vi "tuning_test.vi"() -> ()   [LabVIEW 2011]
panel:
  out "XY Graph":cluster{i32[], dbl[]}(graph)
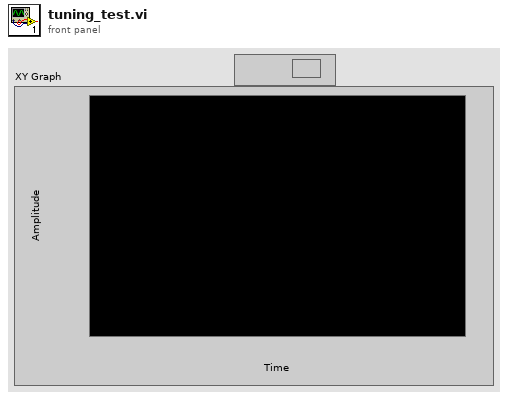
[diagram p1: front panel]
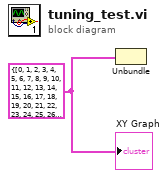
[diagram p0: block diagram]
diagram:
  w1 = cluster{i32[], dbl[]} {[0, 1, 2, 3, 4, 5, 6, 7, 8, 9, 10, 11, 12, 13, 14, 15, 16, 17, 18, 19, 20, 21, 22, 23, 24, 25, 26, 27, 28, 29, 30, 31, 32, 33, 34, 35, 36, 37, 38, 39, 40, 41, 42, 43, 44, 45, 46, 47, 48, 49, 50, 51, 52, 53, 54, 55, 56, 57, 58, 59, 60, 61, 62, 63, 64, 65, 66, 67, 68, 69, 70, 71, 72, 73, 74, 75, 76, 77, 78, 79, 80, 81, 82, 83, 84, 85, 86, 87, 88, 89, 90, 91, 92, 93, 94, 95, 96, 97, 98, 99, 100, 101, 102, 103, 104, 105, 106, 107, 108, 109, 110, 111, 112, 113, 114, 115, 116, 117, 118, 119, 120, 121, 122, 123, 124, 125, 126, 127, 128, 129, 130, 131, 132, 133, 134, 135, 136, 137, 138, 139, 140, 141, 142, 143, 144, 145, 146, 147, 148, 149, 150, 151, 152, 153, 154, 155, 156, 157, 158, 159, 160, 161, 162, 163, 164, 165, 166, 167, 168, 169, 170, 171, 172, 173, 174, 175, 176, 177, 178, 179, 180, 181, 182, 183, 184, 185, 186, 187, 188, 189, 190, 191, 192, 193, 194, 195, 196, 197, 198, 199, 200, 201, 202, 203, 204, 205, 206, 207, 208, 209, 210, 211, 212, 213, 214, 215, 216, 217, 218, 219, 220, 221, 222, 223, 224, 225, 226, 227, 228, 229, 230, 231, 232, 233, 234, 235, 236, 237, 238, 239, 240, 241, 242, 243, 244, 245, 246, 247, 248, 249, 250, 251, 252, 253, 254, 255, 256, 257, 258, 259, 260, 261, 262, 263, 264, 265, 266, 267, 268, 269, 270, 271, 272, 273, 274, 275, 276, 277, 278, 279, 280, 281, 282, 283, 284, 285, 286, 287, 288, 289, 290, 291, 292, 293, 294, 295, 296, 297, 298, 299, 300, 301, 302, 303, 304, 305, 306, 307, 308, 309, 310, 311, 312, 313, 314, 315, 316, 317, 318, 319, 320, 321, 322, 323, 324, 325, 326, 327, 328, 329, 330, 331, 332, 333, 334, 335, 336, 337, 338, 339, 340, 341, 342, 343, 344, 345, 346, 347, 348, 349, 350, 351, 352, 353, 354, 355, 356, 357, 358, 359, 360, 361, 362, 363, 364, 365, 366, 367, 368, 369, 370, 371, 372, 373, 374, 375, 376, 377, 378, 379, 380, 381, 382, 383, 384, 385, 386, 387, 388, 389, 390, 391, 392, 393, 394, 395, 396, 397, 398, 399, 400, 401, 402, 403, 404, 405, 406, 407, 408, 409, 410, 411, 412, 413, 414, 415, 416, 417, 418, 419, 420, 421, 422, 423, 424, 425, 426, 427, 428, 429, 430, 431, 432, 433, 434, 435, 436, 437, 438, 439, 440, 441, 442, 443, 444, 445, 446, 447, 448, 449, 450, 451, 452, 453, 454, 455, 456, 457, 458, 459, 460, 461, 462, 463, 464, 465, 466, 467, 468, 469, 470, 471, 472, 473, 474, 475, 476, 477, 478, 479, 480, 481, 482, 483, 484, 485, 486, 487, 488, 489, 490, 491, 492, 493, 494, 495, 496, 497, 498, 499, 500, 501, 502, 503, 504, 505, 506, 507, 508, 509, 510, 511, 512, 513, 514, 515, 516, 517, 518, 519, 520, 521, 522, 523, 524, 525, 526, 527, 528, 529, 530, 531, 532, 533, 534, 535, 536, 537, 538, 539, 540, 541, 542, 543, 544, 545, 546, 547, 548, 549, 550, 551, 552, 553, 554, 555, 556, 557, 558, 559, 560, 561, 562, 563, 564, 565, 566, 567, 568, 569, 570, 571, 572, 573, 574, 575, 576, 577, 578, 579, 580, 581, 582, 583, 584, 585, 586, 587, 588, 589, 590, 591, 592, 593, 594, 595, 596, 597, 598, 599, 600, 601, 602, 603, 604, 605, 606, 607, 608, 609, 610, 611, 612, 613, 614, 615, 616, 617, 618, 619, 620, 621, 622, 623, 624, 625, 626, 627, 628, 629, 630, 631, 632, 633, 634, 635, 636, 637, 638, 639, 640, 641, 642, 643, 644, 645, 646, 647, 648, 649, 650, 651, 652, 653, 654, 655, 656, 657, 658, 659, 660, 661, 662, 663, 664, 665, 666, 667, 668, 669, 670, 671, 672, 673, 674, 675, 676, 677, 678, 679, 680, 681, 682, 683, 684, 685, 686, 687, 688, 689, 690, 691, 692, 693, 694, 695, 696, 697, 698, 699, 700, 701, 702, 703, 704, 705, 706, 707, 708, 709, 710, 711, 712, 713, 714, 715, 716, 717, 718, 719], [0.005163496779999999, 0.005067374419, 0.005019692889999998, 0.004978500865999999, 0.0049584110729999995, 0.00494455779, 0.004903066485, 0.004896530929, 0.004880330292, 0.004855177923999999, 0.0047993269750000005, 0.0046631170910000005, 0.004542808654000001, 0.004450621223, 0.004386301712, 0.00432218942, 0.004258146137000001, 0.004217115137, 0.0041646011169999995, 0.004128793907, 0.004072965913999999, 0.004036284378999999, 0.004002226237999999, 0.003977994153, 0.003909670723999999, 0.003839253053, 0.003779075738, 0.003699775296, 0.0036282991290000005, 0.0035629671070000007, 0.0034715622649999995, 0.003404113207, 0.003354659746, 0.0033112354810000003, 0.0032005922650000006, 0.003136986193, 0.00301980749, 0.0029431304430000004, 0.0028419683679999997, 0.002778316312, 0.002698302478, 0.0026508510799999998, 0.002591755498, 0.002476762958, 0.002406690456, 0.002356040384, 0.0023017082590000002, 0.002219623326, 0.0021449944, 0.0020812042740000003, 0.002020704862, 0.001944258006, 0.0018612755710000002, 0.001797554502, 0.0017389191200000002, 0.0016755202440000001, 0.001597784644, 0.001522603363, 0.0014572023889999999, 0.001393688319, 0.0013246974999999999, 0.001252392749, 0.0011796738609999998, 0.00110727715, 0.00104031133, 0.0009799039515, 0.0009230175054000001, 0.0008696749981, 0.0008188407983999999, 0.0007630129285000001, 0.0007079674803999999, 0.0006573633814, 0.0006091065414, 0.0005715965176, 0.0005455925944, 0.0005262162478000002, 0.0005116264509000001, 0.0004915136727, 0.00046408299230000003, 0.0004366523296, 0.00042381145470000005, 0.0004150437628, 0.0003989581746, 0.000375784759, 0.00034384366010000003, 0.00030764528780000003, 0.00027413941000000005, 0.0002414158765, 0.0002199223687, 0.0002098199273, 0.00021005008180000002, 0.00021156888669999997, 0.00021182201900000002, 0.0002084162045, 0.0002094287224, 0.00021014211380000004, 0.0002181274147, 0.00022921935309999997, 0.00023499543020000002, 0.00023973596109999997, 0.0002453969951, 0.0002538885048, 0.0002666143584, 0.0002948734793, 0.0003390800908, 0.0003910879545, 0.0004366983632, 0.00047275868710000004, 0.0005059883988, 0.0005384818010999999, 0.0005604355597, 0.0005781550134, 0.0005994874285, 0.0006350644282999999, 0.0006777292814999999, 0.0007130301907, 0.0007522661879, 0.0008017426417, 0.0008465476624000001, 0.0008945282665999999, 0.0009516218445, 0.0010136170074, 0.001077591267, 0.0011420027110000002, 0.001207771943, 0.001281549398, 0.0013521281650000002, 0.001426711048, 0.001501409012, 0.0015786613930000002, 0.0016642902170000001, 0.001764876955, 0.001854556053, 0.0019330509819999997, 0.001988441614, 0.00206979015, 0.002169617591, 0.002259664702, 0.0023309569119999997, 0.002392123616, 0.002458721283, 0.002527873357, 0.00262843708, 0.002727988362, 0.002846892923, 0.002969203446, 0.0030465937679999998, 0.003119519911, 0.0031939186620000004, 0.0032623112420000003, 0.0033096936300000004, 0.003375554829, 0.0034586063109999995, 0.003576659433, 0.0036718844429999994, 0.003751437995, 0.003836882673, 0.003914204169, 0.0039525425990000005, 0.003981192829, 0.004038470564999999, 0.004073679541, 0.00410115607, 0.004147710045, 0.0041927452670000006, 0.004247215295999999, 0.004309003288, 0.0043698708999999995, 0.00441168435, 0.004466361599, 0.004509693895000001, 0.004537032589, 0.004605563264, 0.00467890352, 0.004729944886000001, 0.004770423472, 0.0047632667250000005, 0.004818588309, 0.0048896042619999995, 0.004951392302, 0.005038793154, 0.005045282606999999, 0.005042152991, 0.0050377344239999995, 0.0050650041549999995, 0.005108750517, 0.005150540779999999, 0.005148584815, 0.0051888794160000005, 0.005234305656000001, 0.005266131739999999, 0.00529043288, 0.005290870042, 0.005267558526000001, 0.005254533513999999, 0.005249194707999999, 0.00528870672, 0.005303756894, 0.0053155161440000005, 0.005309855147999999, 0.005336917751, 0.005349045108, 0.005311903311, 0.005294805067, 0.005262058507, 0.005250529385000001, 0.0052575481139999995, 0.005224502552000001, 0.005146951043, 0.005057778255, 0.004995622066999999, 0.004946490797, 0.004906219151, 0.004888568586, 0.004888361552999999, 0.004896485014, 0.0048900875270000005, 0.004875382596, 0.004836514871, 0.004757490522, 0.00467503746, 0.004597578103999999, 0.004487878130999999, 0.004384138528, 0.004336963361, 0.0043169425319999994, 0.004281457513, 0.004219807636, 0.004116298118, 0.004016700945, 0.003940990356, 0.0038744617960000003, 0.0038080253429999995, 0.0037455238859999997, 0.003657731948, 0.003582619737, 0.0035078526250000006, 0.0034235816210000007, 0.0033413816000000007, 0.0032778216060000004, 0.003217046055, 0.003170722258, 0.0031204172869999996, 0.003048411825, 0.002945592673, 0.002855016361, 0.0027618854760000006, 0.0026850243569999997, 0.002612581617, 0.00253312008, 0.00246613128, 0.0024227760489999996, 0.002364439843, 0.0023274590500000003, 0.0022610685320000002, 0.002164946101, 0.002067350922, 0.0019887407769999996, 0.001923454867, 0.001850229654, 0.0017620695070000001, 0.001694459374, 0.0016268951480000002, 0.0015538541120000001, 0.001474392554, 0.001410556398, 0.001351690911, 0.001288291966, 0.001230554061, 0.001174427126, 0.0011069089519999999, 0.001031727705, 0.0009569837246000001, 0.0008908923716, 0.0008290122205, 0.0007700086863, 0.0007149171957999999, 0.0006650035096, 0.0006183804945000001, 0.0005712513230000001, 0.0005292768591000001, 0.0004940450628, 0.0004643591412, 0.0004372506374, 0.00041294963459999996, 0.0003859331977, 0.0003572828487, 0.0003281262587, 0.00029933788179999993, 0.0002788108745, 0.00026277128490000004, 0.00024406230079999998, 0.0002255373766, 0.00020860031510000002, 0.0001933201508, 0.00017527848540000005, 0.00016823673240000002, 0.0001699626187, 0.0001768203073, 0.0001852888322, 0.0001904666091, 0.00019161723450000003, 0.0001907887724, 0.0001927218181, 0.0001992112841, 0.00020358363099999996, 0.00021398521350000002, 0.00022770054620000003, 0.0002466166451, 0.00026771892710000003, 0.0002917667937, 0.00031986484809999995, 0.0003460528416000001, 0.00037293126220000006, 0.0004022719369, 0.0004359389509, 0.00047720006849999994, 0.0005206933186999999, 0.0005615861563000001, 0.0006020648232, 0.0006502986243999999, 0.0007099005335, 0.0007726551091000001, 0.0008327862946999999, 0.0008956559586000001, 0.0009586866014999999, 0.001016723679, 0.0010723444630000001, 0.0011222811769999999, 0.001164969021, 0.0012200374510000001, 0.0012946433980000002, 0.00137817806, 0.001445811289, 0.0015114884359999998, 0.001574979397, 0.001653060223, 0.001743268442, 0.0018260437180000002, 0.001895034629, 0.001958824833, 0.00203018596, 0.002105229162, 0.002169778616, 0.002219945472, 0.002265348843, 0.0023174947370000003, 0.002397439465, 0.002500258503, 0.002580778578, 0.0026439934290000003, 0.0027078756369999994, 0.0028000168490000003, 0.0028692149090000004, 0.0029648310740000004, 0.0030518636099999994, 0.0031166893659999996, 0.0031846676739999994, 0.0032518175889999995, 0.003347433826, 0.003455821797, 0.003553877281, 0.003617621354, 0.003675336319999999, 0.00374349875, 0.0038037910130000003, 0.003868041328999999, 0.003943475755, 0.004014146561999999, 0.004046340846, 0.004107139305, 0.0041663730509999995, 0.0042568343699999995, 0.004356063435999999, 0.0044169541909999995, 0.0044630248559999995, 0.004542509419, 0.004655016772000001, 0.004711304979, 0.004742808825, 0.004761793882000001, 0.0047857495969999995, 0.004832510696000001, 0.00492881732, 0.0049911807310000006, 0.0050461341630000005, 0.005067282403000001, 0.005071516567000001, 0.00507338061, 0.005063347284, 0.005069054336, 0.005091767478, 0.005116666806, 0.005122028617, 0.005140737817, 0.005161931925000001, 0.005183379492, 0.005233638315, 0.005237021204, 0.005229266126999999, 0.005247606896999999, 0.005280261392, 0.0052912842039999994, 0.005279778131, 0.005226550624, 0.005188304094, 0.005178178661, 0.0051268381989999995, 0.005104355094, 0.005108704605, 0.005076901521, 0.005056282458999999, 0.005045949994, 0.004990398185, 0.004914710716999999, 0.004886566662, 0.004869537615, 0.004838931233999999, 0.004827125882999999, 0.004853613023, 0.004844177930999999, 0.0048127660039999996, 0.004760919464, 0.004721683404, 0.004676740431, 0.004602088361, 0.004554452888000001, 0.004508612305000001, 0.004448849336, 0.004371596872, 0.004298141598, 0.004235801287, 0.004205908252, 0.004187636310000001, 0.0041415197299999994, 0.004125963336, 0.004063507961, 0.003969249547, 0.0038744617950000003, 0.003814123547, 0.0037748644130000003, 0.0036916290170000005, 0.0036297949269999998, 0.003543337715, 0.0034873716999999998, 0.003408899716, 0.0033433146770000003, 0.0032485729079999998, 0.0031890631200000006, 0.00310387148, 0.0030086235609999997, 0.00292709088, 0.002862150221, 0.002791617323, 0.002713996939, 0.0026494703480000005, 0.0025744732, 0.0024894427510000006, 0.002392468835, 0.002292365233, 0.002199303521, 0.002107852535, 0.002036353295, 0.001962161554, 0.0018770160160000004, 0.001794470871, 0.0017097855120000002, 0.001611223816, 0.001543613592, 0.00148196359, 0.001423236228, 0.001358341518, 0.001293032534, 0.001222062565, 0.001159607119, 0.0010932856929999999, 0.0010236963872, 0.0009635652298000001, 0.0009028587725, 0.000857639557, 0.0008077258304000001, 0.0007566845511000001, 0.0007070009772, 0.0006628863455, 0.0006217633317, 0.0005855880094999999, 0.0005464441142, 0.0005036641901, 0.00046233404729999997, 0.0004282298411, 0.00039603559980000007, 0.0003605506209, 0.00032757394370000004, 0.000304515616, 0.00028373550739999997, 0.0002713549037, 0.0002596646256, 0.0002497693291, 0.0002355247037, 0.0002155960598, 0.00019587451529999998, 0.0001770734408, 0.000159054788, 0.0001439126571, 0.00013440858750000002, 0.0001292998684, 0.00012545681080000003, 0.000125709966, 0.00012743586850000001, 0.00013588138679999998, 0.0001566384904, 0.0001995334691, 0.00025066682289999996, 0.0002854384305, 0.0003082436045, 0.0003360424948, 0.00036229956, 0.000381583866, 0.0004054016084000001, 0.0004310603923, 0.0004553843549, 0.00048244685159999997, 0.0005036872405, 0.0005258480787000001, 0.0005511846274999999, 0.0005961046437999999, 0.0006541646784999999, 0.0007094862638, 0.0007599062577000001, 0.0008092907257000001, 0.0008690306511000001, 0.0009344316145, 0.0009934812493, 0.0010433259299999999, 0.001086013754, 0.001130910742, 0.0011782931620000002, 0.0012328553359999999, 0.001308726915, 0.001378408237, 0.001444637638, 0.0015097855019999998, 0.0015721488500000003, 0.001642727667, 0.00171065994, 0.0017643017220000002, 0.001836790504, 0.0019079906049999998, 0.001984391478, 0.002053635497, 0.0021220741330000006, 0.002211799169, 0.0022944133749999997, 0.0023712745169999997, 0.0024567881589999995, 0.002509371379, 0.002560458681, 0.0026346044139999997, 0.0027116956900000004, 0.002782550501, 0.002870526583, 0.002963358327, 0.0030565351929999996, 0.0031379067329999994, 0.0032162407179999997, 0.0032958402300000003, 0.003362207835, 0.003419692513, 0.0034609535930000004, 0.0035358586589999998, 0.0036595038600000006, 0.0037571680260000003, 0.003812420623999999, 0.003873633384, 0.0039343629050000006, 0.004006299377, 0.0040949428449999995, 0.004153969373, 0.004222154711, 0.004285415634, 0.0043417268920000005, 0.004374473357, 0.004444177728, 0.0045582499350000005, 0.0046384708939999995, 0.0046693995129999995, 0.00467989319, 0.004701041338000001, 0.004724030662, 0.004774105594000001, 0.004809222417000001, 0.004851127648, 0.004924030649, 0.0049912726049999995, 0.005023006677, 0.005077914055999999, 0.005120693984, 0.005134317186, 0.005104194067999999, 0.005083690072, 0.00509416056, 0.005126377987, 0.005150586879000001, 0.005199188876999999, 0.005219301722, 0.005296830229, 0.005336526360999999, 0.005388143099999999, 0.005415435507, 0.005421695065000001, 0.005405218294999999, 0.005341404956, 0.005274968455000001, 0.005228736671000001, 0.0052153436, 0.005189569852, 0.005208048643, 0.005241669668, 0.005276855594999999, 0.005281527062, 0.0052899036100000005, 0.005275451763999999, 0.005268248869, 0.005240703094, 0.0051826431410000005, 0.005091099952, 0.004989569772999999, 0.004953141277, 0.004948745902, 0.0049368715850000005, 0.004900673265999999, 0.004811661551, 0.004722051603, 0.004648021049, 0.004624617566, 0.004587935795, 0.004572908812, 0.004556961263999999, 0.004521522300000001, 0.004465671256, 0.004398705346, 0.004334869049, 0.004289028701999998, 0.004215849563, 0.004108957434, 0.004019669535000001, 0.003954866830000001, 0.003871585266, 0.003780916776, 0.0036860139809999997, 0.003617621282, 0.00356038972, 0.0034921122489999998, 0.003410602663, 0.0033202333139999997, 0.0032416922730000007, 0.003172402177, 0.003135375354, 0.003090041201, 0.0030290355669999997, 0.0029374694689999993, 0.0028474683649999995, 0.002758180491, 0.002666269383, 0.0025817221250000006, 0.002504446778, 0.002439229842, 0.002370423031, 0.002290064027, 0.0022110397, 0.002142025855, 0.0020690537520000004, 0.001996772121, 0.0019149633240000002, 0.0018385164199999997, 0.0017613330990000002, 0.001678972003, 0.0016000398789999999, 0.001528126291, 0.001461068449, 0.0013989351800000002, 0.00133981657, 0.001274346571, 0.0012160793649999997, 0.001157996304, 0.001106724843, 0.0010690997119999998, 0.001026757038, 0.0009805482986, 0.0009268145599999999, 0.0008769929002, 0.0008318657986999999, 0.0007825733861, 0.000738573825, 0.0006929634545999999, 0.0006484806479999999, 0.0006041589366999999, 0.0005599523195, 0.000515078305, 0.0004700201856, 0.0004239035189, 0.0003822972503, 0.00034029977099999997, 0.0003029507847, 0.00027239044139999995, 0.000245120858, 0.00022084285170000003, 0.0002084392081, 0.0001973932944, 0.0001852427944, 0.00016885804800000003, 0.00015291049060000002, 0.0001452013573, 0.00014220980519999999, 0.0001393102299, 0.0001426240007, 0.0001503561419, 0.00015682259099999998, 0.0001718726562, 0.000191272024]} ("XY Graph")
  n1 = Unbundle(w1) -> ()  [unwired: 2 out]
  "XY Graph" <- w1
